vi "Read Return DER_Info Msg.vi"(11 "EMS Generic in":refnum<class "EMS Generic.lvclass">) -> (2 "Return DER_Info Msg":refnum<class "Return DER_Info Msg.lvclass">, 3 "EMS Generic out":refnum<class "EMS Generic.lvclass">)   [LabVIEW 2018, in "EMS Generic Actor.lvlib" / "EMS Generic.lvclass"]
uses:
  EMS Generic.lvclass
  EMS Generic Messages/Return DER_Info Msg/Return DER_Info Msg.lvclass
  EMS Generic.lvclass/EMS Generic.ctl
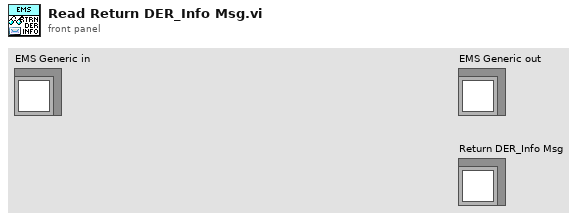
[diagram p1: front panel]
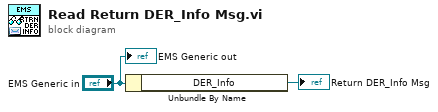
[diagram p0: block diagram]
diagram:
  n1 = Unbundle By Name("EMS Generic in") -> ("DER_Info"=→"Return DER_Info Msg":refnum<class "Return DER_Info Msg.lvclass">)
  "EMS Generic out" <- "EMS Generic in"
